vi "GetNameList.vi"(8 "error in (no error)":errorcluster, 11 "Devices":refnum<class "Device.lvclass">[](array[class])) -> (0 "error out":errorcluster, 2 "Names in use":string[](array[string]), 3 "Devices out":refnum<class "Device.lvclass">[](array[class]))   [LabVIEW 2013]
doc: "Returns array of device names, in order of device array."
uses:
  Device/Device.lvclass
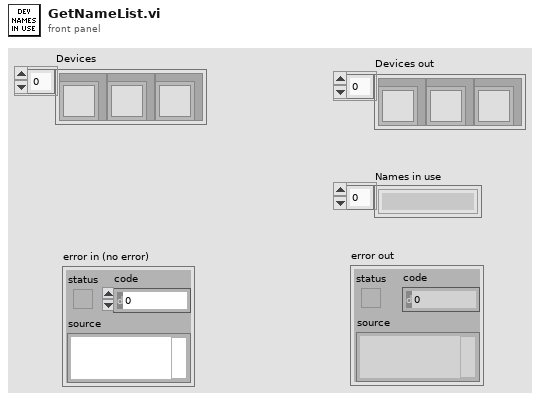
[diagram p1: front panel]
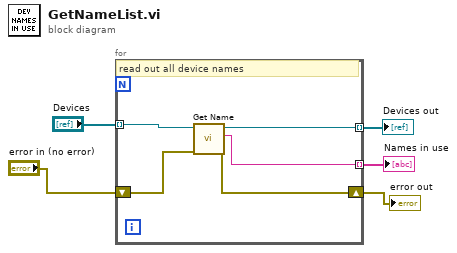
[diagram p0: block diagram]
diagram:
  n1 = for {
    tunnel: "Devices" -> [w10] mode=indexing
    tunnel: [w9] -> w4 mode=indexing
    tunnel: [w8] -> w3 mode=indexing
    shift-right: [w6] -> w1
    shift-left: "error in (no error)" -> [w7]
    # "read out all device names"
    n2 = call-dynamic "Get Name.vi"("error in (no error)"=w7, "Device in"=w10) -> ("error out"=w6:errorcluster, "Name"=w8:string, "Device out"=w9:refnum<class "Device.lvclass">)  [unwired: 7 in]
  }
  "Devices out" <- w4
  "Names in use" <- w3
  "error out" <- w1
